vi "NXT_MIDBRAIN Check Max Weight Behavior.vi"(1 "Behavior #":i32, 2 "_behaviorWeights":T1) -> (0 "Max?":bool)   [LabVIEW 2012, in "Tugboat.lvrbt"]
uses:
  Tugboat.lvrbt
  behaviorWeights_t.ctl
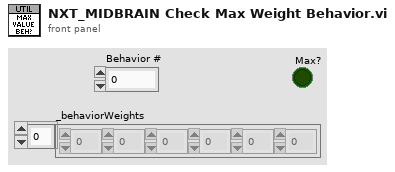
[diagram p1: front panel]
types:
  T1 = typedef "behaviorWeights_t.ctl" = i8[]
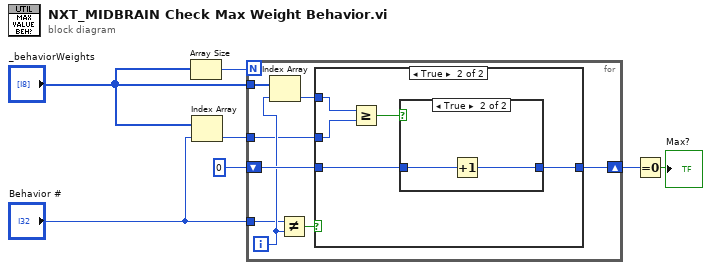
[diagram p0: block diagram]
diagram:
  n1 = Array Size(array="_behaviorWeights") -> (size(s)=w1:i32)
  n2 = Index Array(array="_behaviorWeights", index="Behavior #") -> (element=w5:i8)
  n3 = for {
    N: w1 -> [_]
    shift-right: [w14] -> w6
    shift-left: i8 0 -> [w13]
    tunnel: "Behavior #" -> [w9]
    tunnel: "_behaviorWeights" -> [w12]
    tunnel: w5 -> [w8]
    i -> [w11]
    n4 = Index Array(array=w12, index=w11) -> (element=w10:i8)
    n5 = Not Equal?(x=w9, y=w11) -> (x != y?=w15:bool)
    n6 = case shown="True" w15 {
      tunnel: [w16 w17] -> w14
      tunnel: w13 -> [w16 w18]
      tunnel: w10 -> [_ w21]
      tunnel: w8 -> [_ w20]
      frame False {
      }
      frame True {
        n7 = Greater Or Equal?(x=w21, y=w20) -> (x >= y?=w19:bool)
        n8 = case shown="True" w19 {
          tunnel: w18 -> [w22 w24]
          tunnel: [w22 w23] -> w17
          frame False {
          }
          frame True {
            n9 = Increment(x=w24) -> (x+1=w23:i8)
          }
        }
      }
    }
  }
  n10 = Equal To 0?(x=w6) -> (x = 0?=→"Max?":bool)
